vi "手动5界面.vi"(8 "错误输入（无错误）":errorcluster, 10 "界面切换队列":refnum<queue>, 11 "VISA资源名称输入":refnum<visa-resource-name>) -> (0 "错误输出":errorcluster, 3 "VISA资源名称输出":refnum<visa-resource-name>)   [LabVIEW 2018]
panel:
  out "R3":bool
  out "毫秒计时值":u32
  in  "枚举":T1(ring)
  in  "选项卡控件":enum32{"选项卡 1", "选项卡 2"}(tab)
  out "写R14A+读R14B+Z2下降取料":bool
  out "写R144+读R145+Z1下降取料":bool
  out "写R2E+读Y1C+2号吸嘴真空":bool
  out "写R2C+读Y1B+1号吸嘴真空":bool
  out "写R66+读R67+Z2下降取料":bool
  out "写R62+读R63+Z1下降取料":bool
  out "写R1F+读R5F+R2轴旋转定位":bool
  out "写R1C+读R5C+R1轴旋转定位":bool
  out "写R6C+读R6D+Z轴校正位取料":bool
  out "写R64+读R65+XYZ2到2号飞达位":bool
  out "写R60+读R61+XYZ1到飞达位":bool
  out "写R6A+读R6B+Z轴校正位放料":bool
  out "写R3F+读R4F+Z2下降编带":bool
  out "写R3D+读R4D+Z1下降编带":bool
  out "写R148+读R149+Z2下降放料":bool
  out "写R168+读R168+切换+快速":bool
  out "写R142+读R143+Z1下降放料":bool
  out "写R68+读R69+XY到校正位":bool
  out "写R3E+读R4E+XYZ2到2号编带位":bool
  out "写R3C+读R4C+XYZ1到1号编带位":bool
  out "写R146+读R147+XYZ2到烧录位":bool
  out "手动4界面":bool
  out "DDT90356":dbl
  out "DDT90348":dbl
  out "自动界面":bool
  out "手动界面":bool
  out "参数界面":bool
  out "IO界面":bool
  out "产品界面":bool
  out "字符串":string
  out "DDT90352":dbl
  out "DDT90360":dbl
  out "DT1184":T2(ring)
  out "写R0+读R1+手动启动":bool
  out "写R4+读R4+手动停止":bool
  out "写R8+读R9+机器复位":bool
  out "写R80+读R80+报警清除":bool
  out "烧录座手动界面":bool
  out "通讯周期":dbl
  in  "DT62+枚举":enum16{"90度", "180度", "270度"}(ring)
  in  "DT63+枚举":enum16{"90度", "180度", "270度"}(ring)
  out "写R81+读R81+切换+快速":bool
  out "写R140+读141+XYZ1到烧录位":bool
  out "写DT120+指定烧录编号":dbl
  # "X"
  # "Z1"
  # "Z2"
  # "Y"
  # "指定烧录编号"
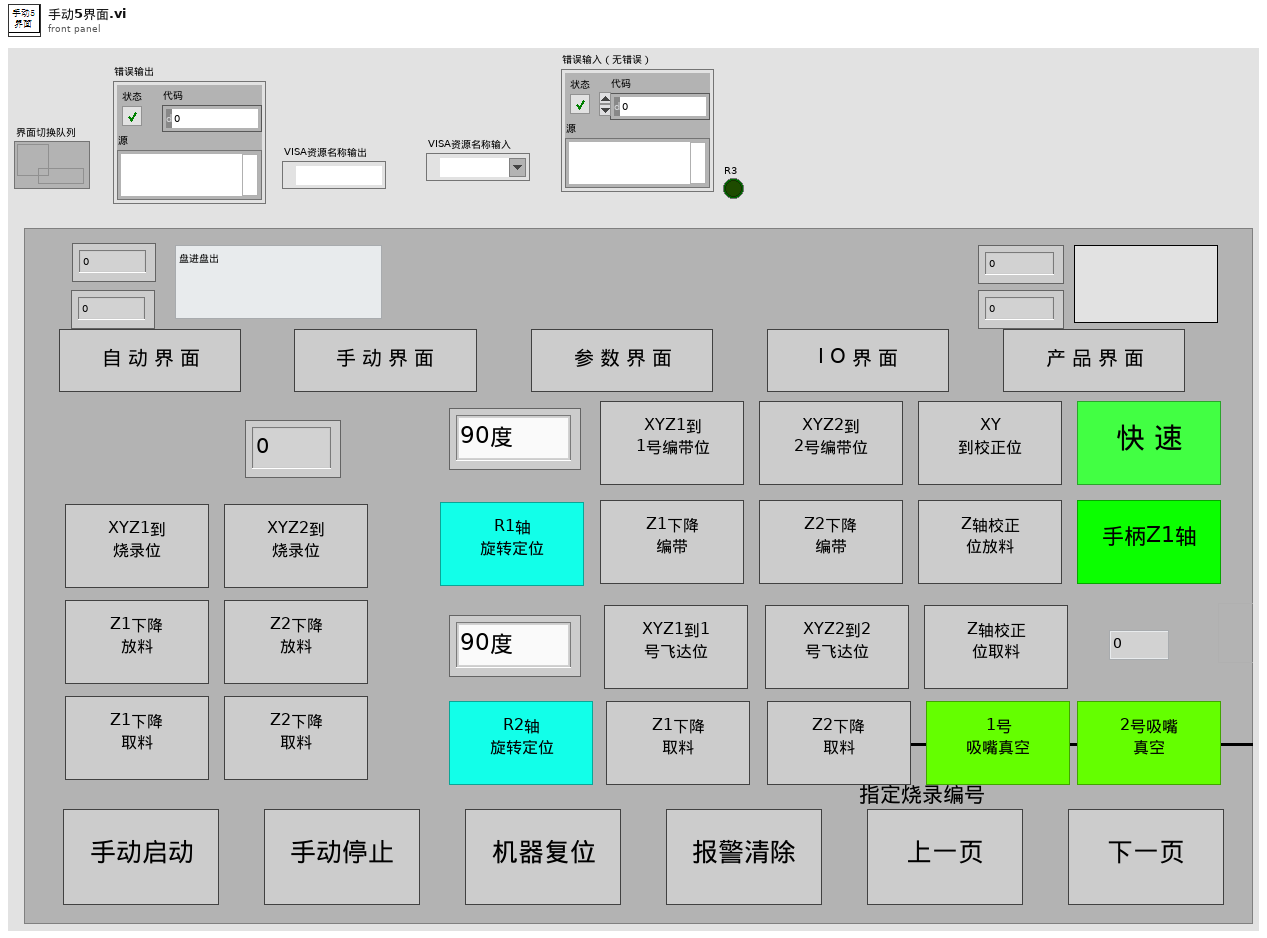
[diagram p1: front panel]
types:
  T1 = enum16{"读初始化", "读R149+8", "读R141+8", "读R4C+8", "读R61+8", "读R77+8", "读R168+8", "读Y1B+8", "读R80+8", "读R69+8", "读R5C+8", "读R9+8", "读R1+8", "读DT770+10", "读DDT604+5", "读DT1184", "读DT62+10", "读DDT90356", "读DDT90348", ""}
  T2 = enum16{"盘进盘出", "卷进卷出", "盘进卷出", "管进盘出", "管进卷出", "卷进盘出", ""}
  T3 = typedef "数据簇.ctl" = cluster{"字符串":string, "数值":i32, "布尔":bool}
  T4 = enum8{"Enabled", "Disabled", "Disabled and Grayed Out"}
  T5 = typedef "lveventtype.ctl" = enum32{"Null", "Timeout", "Annotation Menu Selection", "Annotation Menu Selection?", "App Instance Close", "App Instance Close?", "Autoscale Range Change", "Bookmark Info Change", "Cell Edit", "Cell Edit?", "Cursor Grab", "Cursor Grab?", "Cursor Menu Selection", "Cursor Menu Selection?", "Cursor Move", "Cursor Release", "Data Change", "Direction Change", "Display State Change", "Drag Ended", "Drag Enter", "Drag Leave", "Drag Over", "Drag Source Update", "Drag Starting", "Drag Starting?", "Drop", "Exec State Change", "Key Down", "Key Down?", "Key Repeat", "Key Repeat?", "Key Up", "Listbox Double Click", "Menu Activation?", "Menu Selection (App)", "Menu Selection? (App)", "Menu Selection (User)", "Mouse Down", "Mouse Down?", "Mouse Enter", "Mouse Leave", "Mouse Move", "Mouse Up", "Mouse Wheel", "NI Security User Change (App)", "Pane Size", "Panel Close", "Panel Close?", "Panel Resize", "Plot Attribute Change", "Scale Range Change", "Shortcut Menu Activation?", "Shortcut Menu Selection (App)", "Shortcut Menu Selection? (App)", "Shortcut Menu Selection (User)", "Tree Double Click", "Tree Drag", "Tree Drag?", "Tree Drop", "Tree Drop?", "Tree Item Close", "Tree Item Close?", "Tree Item Open", "Tree Item Open?", "User Event", "Value Change"}
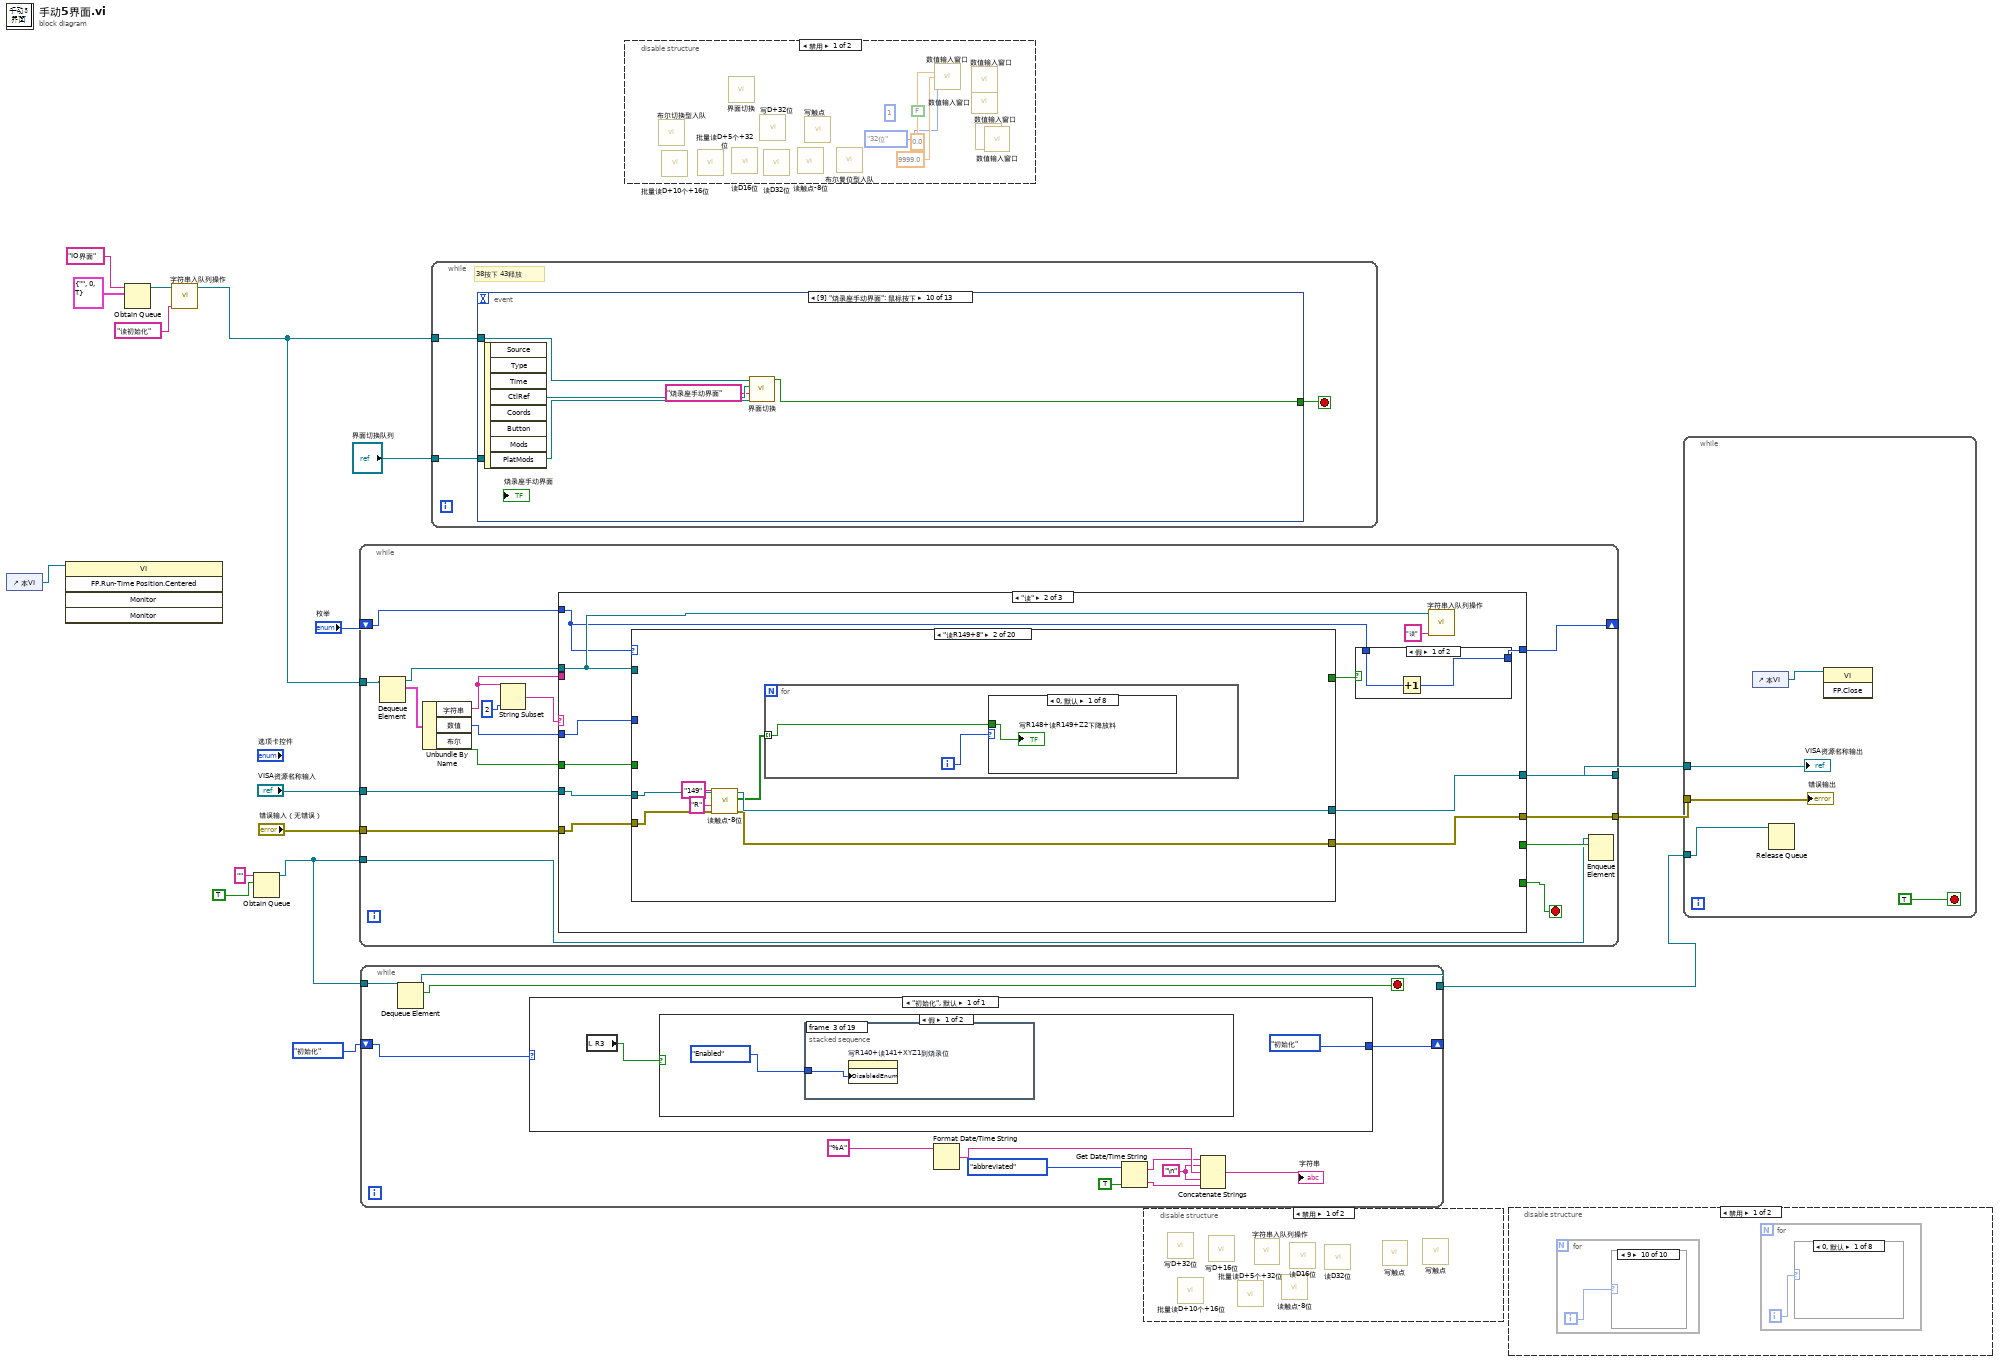
[diagram p0: block diagram]
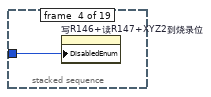
[diagram p4: hidden frame]
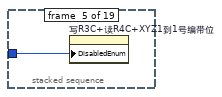
[diagram p5: hidden frame]
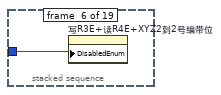
[diagram p6: hidden frame]
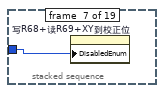
[diagram p7: hidden frame]
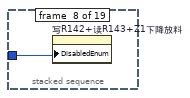
[diagram p8: hidden frame]
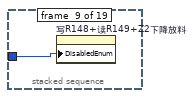
[diagram p9: hidden frame]
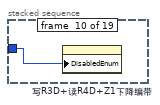
[diagram p10: hidden frame]
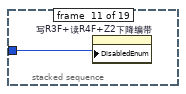
[diagram p11: hidden frame]
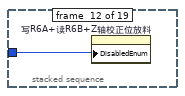
[diagram p12: hidden frame]
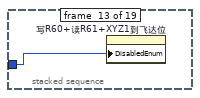
[diagram p13: hidden frame]
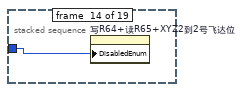
[diagram p14: hidden frame]
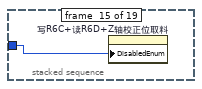
[diagram p15: hidden frame]
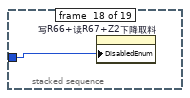
[diagram p18: hidden frame]
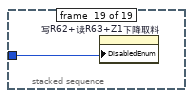
[diagram p19: hidden frame]
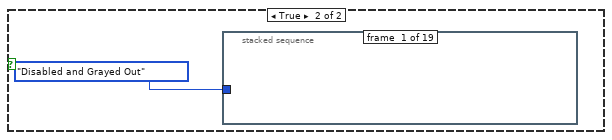
[diagram p20: hidden frame]
diagram:
  n1 = control-ref of="本VI"() -> (w2:refnum<vi>)
  n2 = invoke class="VI" method="FP.Run-Time Position.Centered"(reference=w2) -> ()  [unwired: 4 in, 5 out]
  n3 = Obtain Queue(name (unnamed)="IO界面" ("名称（未命名）"), element data type=T3 {"字符串"="", "数值"=0, "布尔"=TRUE}) -> (queue out=w10:refnum<queue>)  [unwired: 3 in, 2 out]
  n4 = call "字符串入队列操作.vi"("字符消息入队列"="读初始化", "界面切换队列"=w10) -> ("队列输出"=w3:refnum<queue>)  [unwired: 9 in]
  n5 = Obtain Queue(name (unnamed)="" ("名称（未命名）"), element data type=TRUE) -> (queue out=w6:refnum<queue>)  [unwired: 3 in, 2 out]
  n6 = while {
    tunnel: w3 -> [w34]
    tunnel: "VISA资源名称输入" -> [w27]
    tunnel: "错误输入（无错误）" -> [w26]
    tunnel: [w25] -> w12
    tunnel: [w24] -> w11
    shift-right: [w21] -> _
    shift-left: "枚举" -> [w22]
    tunnel: w6 -> [w18]
    stop <- w20 stop-if-true
    n7 = Dequeue Element(queue=w34) -> (queue out=w31:refnum<queue>, element=w33:T3)  [unwired: 2 in, 2 out]
    n8 = Unbundle By Name(w33) -> ("字符串"=w28:string, "数值"=w30:i32, "布尔"=w29:bool)
    n9 = String Subset(string=w28, length (rest)=2 ("长度（剩余）")) -> (substring=w32:string)  [unwired: 1 in]
    n10 = case shown="\"读\"" w32 {
      selector: w32 -> [w37 _ _]
      tunnel: w31 -> [_ w45 w277]
      tunnel: w30 -> [_ w52 w276]
      tunnel: w29 -> [_ w51 w275]
      tunnel: w28 -> [_ _ w269]
      tunnel: w27 -> [w36 w50 w274]
      tunnel: w26 -> [w35 w49 w273]
      tunnel: [w36 w48 w271] -> w25
      tunnel: [w35 w47 w270] -> w24
      tunnel: [_ _ w272] -> w20
      tunnel: w22 -> [_ w43 _]
      tunnel: [_ w42 _] -> w21
      tunnel: [_ _ w267] -> w19
      frame "", Default {
        n11 = Concatenate Strings("无对应消息分支**" ("消息"), w37, "**" ("字符串"), "读写状态机" ("字符串")) -> (w39:string)
        n12 = One Button Dialog(message=w39) -> ()  [unwired: 1 in, 1 out]
      }
      frame "读" {
        n13 = case shown="\"读R149+8\"" w43 {
          tunnel: w45 -> [_ _ _ _ _ _ _ _ _ _ _ _ _ _ _ _ _ _ _ _]
          tunnel: w52 -> [_ _ _ _ _ _ _ _ _ _ _ _ _ _ _ _ _ _ _ _]
          tunnel: w50 -> [w57 w64 w75 w88 w101 w114 w123 w133 w144 w155 w167 w178 w188 w200 w208 w215 w222 w238 w254 w266]
          tunnel: w49 -> [w56 w63 w74 w87 w100 w113 w122 w132 w143 w154 w166 w177 w187 w199 w207 w214 w221 w237 w253 w265]
          tunnel: [w57 w62 w71 w84 w99 w112 w121 w129 w142 w153 w165 w176 w186 w197 w205 w213 w219 w236 w252 w266] -> w48
          tunnel: [w56 w61 w70 w83 w98 w111 w120 w128 w141 w152 w164 w175 w185 w196 w204 w212 w218 w235 w251 w265] -> w47
          tunnel: w51 -> [_ _ _ _ _ _ _ _ _ _ _ _ _ _ _ _ _ _ _ _]
          tunnel: [_ _ _ _ _ _ _ _ _ _ _ _ _ _ _ _ _ _ _ TRUE] -> w44
          frame "读初始化" {
            n14 = Tick Count (ms)() -> (millisecond timer value=→"毫秒计时值":u32)
          }
          frame "读R149+8" {
            n15 = call "读触点-8位.vi"("error out"=w63, "触点类型"="R", "读取起始地址"="149", "VISA resource name out"=w64) -> ("error IO"=w61:errorcluster, "读取布尔数组"=w58:bool[], "VISA resource name out 2"=w62:refnum<visa-resource-name>)  [unwired: 4 in, 1 out]
            n16 = for {
              tunnel: w58 -> [w65] mode=indexing
              i -> [w66]
              n17 = case shown="0, 默认" w66 {
                tunnel: w65 -> [w67 _ w68 _ _ _ _ _]
                frame 0, Default {
                  "写R148+读R149+Z2下降放料" <- w67
                }
                frame 1 {
                }
                frame 2 {
                  "写R14A+读R14B+Z2下降取料" <- w68
                }
                frame 3 {
                }
                frame 4 {
                }
                frame 5 {
                }
                frame 6 {
                }
                frame 7 {
                }
              }
            }
          }
          frame "读R141+8" {
            n18 = call "读触点-8位.vi"("error out"=w74, "触点类型"="R", "读取起始地址"="141", "VISA resource name out"=w75) -> ("error IO"=w70:errorcluster, "读取布尔数组"=w69:bool[], "VISA resource name out 2"=w71:refnum<visa-resource-name>)  [unwired: 4 in, 1 out]
            n19 = for {
              tunnel: w69 -> [w76] mode=indexing
              i -> [w77]
              n20 = case shown="4" w77 {
                tunnel: w76 -> [w78 _ w79 _ w80 _ w81 _]
                frame 0, Default {
                  "写R140+读141+XYZ1到烧录位" <- w78
                }
                frame 1 {
                }
                frame 2 {
                  "写R142+读R143+Z1下降放料" <- w79
                }
                frame 3 {
                }
                frame 4 {
                  "写R144+读R145+Z1下降取料" <- w80
                }
                frame 5 {
                }
                frame 6 {
                  "写R146+读R147+XYZ2到烧录位" <- w81
                }
                frame 7 {
                }
              }
            }
          }
          frame "读R4C+8" {
            n21 = call "读触点-8位.vi"("error out"=w87, "触点类型"="R", "读取起始地址"="4C", "VISA resource name out"=w88) -> ("error IO"=w83:errorcluster, "读取布尔数组"=w82:bool[], "VISA resource name out 2"=w84:refnum<visa-resource-name>)  [unwired: 4 in, 1 out]
            n22 = for {
              tunnel: w82 -> [w89] mode=indexing
              i -> [w90]
              n23 = case shown="3" w90 {
                tunnel: w89 -> [w91 w92 w93 w94 _ _ _ _]
                frame 0, Default {
                  "写R3C+读R4C+XYZ1到1号编带位" <- w91
                }
                frame 1 {
                  "写R3D+读R4D+Z1下降编带" <- w92
                }
                frame 2 {
                  "写R3E+读R4E+XYZ2到2号编带位" <- w93
                }
                frame 3 {
                  "写R3F+读R4F+Z2下降编带" <- w94
                }
                frame 4 {
                }
                frame 5 {
                }
                frame 6 {
                }
                frame 7 {
                }
              }
            }
          }
          frame "读R61+8" {
            n24 = call "读触点-8位.vi"("error out"=w100, "触点类型"="R", "读取起始地址"="61", "VISA resource name out"=w101) -> ("error IO"=w98:errorcluster, "读取布尔数组"=w95:bool[], "VISA resource name out 2"=w99:refnum<visa-resource-name>)  [unwired: 4 in, 1 out]
            n25 = for {
              tunnel: w95 -> [w102] mode=indexing
              i -> [w103]
              n26 = case shown="6" w103 {
                tunnel: w102 -> [w104 _ w105 _ w106 _ w107 _]
                frame 0, Default {
                  "写R60+读R61+XYZ1到飞达位" <- w104
                }
                frame 1 {
                }
                frame 2 {
                  "写R62+读R63+Z1下降取料" <- w105
                }
                frame 3 {
                }
                frame 4 {
                  "写R64+读R65+XYZ2到2号飞达位" <- w106
                }
                frame 5 {
                }
                frame 6 {
                  "写R66+读R67+Z2下降取料" <- w107
                }
                frame 7 {
                }
              }
            }
          }
          frame "读R77+8" {
            n27 = call "读触点-8位.vi"("error out"=w113, "触点类型"="R", "读取起始地址"="77", "VISA resource name out"=w114) -> ("error IO"=w111:errorcluster, "读取布尔数组"=w108:bool[], "VISA resource name out 2"=w112:refnum<visa-resource-name>)  [unwired: 4 in, 1 out]
            n28 = for {
              tunnel: w108 -> [w115] mode=indexing
              i -> [w116]
              n29 = case shown="0, 默认" w116 {
                tunnel: w115 -> [_ _ _ _ _ _ _ _]
                frame 0, Default {
                }
                frame 1 {
                }
                frame 2 {
                }
                frame 3 {
                }
                frame 4 {
                }
                frame 5 {
                }
                frame 6 {
                }
                frame 7 {
                }
              }
            }
          }
          frame "读R168+8" {
            n30 = call "读触点-8位.vi"("error out"=w122, "触点类型"="R", "读取起始地址"="168", "VISA resource name out"=w123) -> ("error IO"=w120:errorcluster, "读取布尔数组"=w117:bool[], "VISA resource name out 2"=w121:refnum<visa-resource-name>)  [unwired: 4 in, 1 out]
            n31 = for {
              tunnel: w117 -> [w124] mode=indexing
              i -> [w125]
              n32 = case shown="0, 默认" w125 {
                tunnel: w124 -> [w126 _ _ _ _ _ _ _]
                frame 0, Default {
                  "写R168+读R168+切换+快速" <- w126
                }
                frame 1 {
                }
                frame 2 {
                }
                frame 3 {
                }
                frame 4 {
                }
                frame 5 {
                }
                frame 6 {
                }
                frame 7 {
                }
              }
            }
          }
          frame "读Y1B+8" {
            n33 = call "读触点-8位.vi"("error out"=w132, "触点类型"="Y", "读取起始地址"="1B", "VISA resource name out"=w133) -> ("error IO"=w128:errorcluster, "读取布尔数组"=w127:bool[], "VISA resource name out 2"=w129:refnum<visa-resource-name>)  [unwired: 4 in, 1 out]
            n34 = for {
              tunnel: w127 -> [w134] mode=indexing
              i -> [w135]
              n35 = case shown="1" w135 {
                tunnel: w134 -> [w136 w137 _ _ _ _ _ _]
                frame 0, Default {
                  "写R2C+读Y1B+1号吸嘴真空" <- w136
                }
                frame 1 {
                  "写R2E+读Y1C+2号吸嘴真空" <- w137
                }
                frame 2 {
                }
                frame 3 {
                }
                frame 4 {
                }
                frame 5 {
                }
                frame 6 {
                }
                frame 7 {
                }
              }
            }
          }
          frame "读R80+8" {
            n36 = call "读触点-8位.vi"("error out"=w143, "触点类型"="R", "读取起始地址"="80", "VISA resource name out"=w144) -> ("error IO"=w141:errorcluster, "读取布尔数组"=w138:bool[], "VISA resource name out 2"=w142:refnum<visa-resource-name>)  [unwired: 4 in, 1 out]
            n37 = for {
              tunnel: w138 -> [w145] mode=indexing
              i -> [w146]
              n38 = case shown="1" w146 {
                tunnel: w145 -> [w147 w148 _ _ _ _ _ _]
                frame 0, Default {
                  "写R80+读R80+报警清除" <- w147
                }
                frame 1 {
                  "写R81+读R81+切换+快速" <- w148
                }
                frame 2 {
                }
                frame 3 {
                }
                frame 4 {
                }
                frame 5 {
                }
                frame 6 {
                }
                frame 7 {
                }
              }
            }
          }
          frame "读R69+8" {
            n39 = call "读触点-8位.vi"("error out"=w154, "触点类型"="R", "读取起始地址"="69", "VISA resource name out"=w155) -> ("error IO"=w152:errorcluster, "读取布尔数组"=w151:bool[], "VISA resource name out 2"=w153:refnum<visa-resource-name>)  [unwired: 4 in, 1 out]
            n40 = for {
              tunnel: w151 -> [w156] mode=indexing
              i -> [w157]
              n41 = case shown="4" w157 {
                tunnel: w156 -> [w158 _ w159 _ w160 _ _ _]
                frame 0, Default {
                  "写R68+读R69+XY到校正位" <- w158
                }
                frame 1 {
                }
                frame 2 {
                  "写R6A+读R6B+Z轴校正位放料" <- w159
                }
                frame 3 {
                }
                frame 4 {
                  "写R6C+读R6D+Z轴校正位取料" <- w160
                }
                frame 5 {
                }
                frame 6 {
                }
                frame 7 {
                }
              }
            }
          }
          frame "读R5C+8" {
            n42 = call "读触点-8位.vi"("error out"=w166, "触点类型"="R", "读取起始地址"="5C", "VISA resource name out"=w167) -> ("error IO"=w164:errorcluster, "读取布尔数组"=w163:bool[], "VISA resource name out 2"=w165:refnum<visa-resource-name>)  [unwired: 4 in, 1 out]
            n43 = for {
              tunnel: w163 -> [w168] mode=indexing
              i -> [w169]
              n44 = case shown="3" w169 {
                tunnel: w168 -> [w170 _ _ w171 _ _ _ _]
                frame 0, Default {
                  "写R1C+读R5C+R1轴旋转定位" <- w170
                }
                frame 1 {
                }
                frame 2 {
                }
                frame 3 {
                  "写R1F+读R5F+R2轴旋转定位" <- w171
                }
                frame 4 {
                }
                frame 5 {
                }
                frame 6 {
                }
                frame 7 {
                }
              }
            }
          }
          frame "读R9+8" {
            n45 = call "读触点-8位.vi"("error out"=w177, "触点类型"="R", "读取起始地址"="9", "VISA resource name out"=w178) -> ("error IO"=w175:errorcluster, "读取布尔数组"=w172:bool[], "VISA resource name out 2"=w176:refnum<visa-resource-name>)  [unwired: 4 in, 1 out]
            n46 = for {
              tunnel: w172 -> [w179] mode=indexing
              i -> [w180]
              n47 = case shown="0, 默认" w180 {
                tunnel: w179 -> [w181 _ _ _ _ _ _ _]
                frame 0, Default {
                  "写R8+读R9+机器复位" <- w181
                }
                frame 1 {
                }
                frame 2 {
                }
                frame 3 {
                }
                frame 4 {
                }
                frame 5 {
                }
                frame 6 {
                }
                frame 7 {
                }
              }
            }
          }
          frame "读R1+8" {
            n48 = call "读触点-8位.vi"("error out"=w187, "触点类型"="R", "读取起始地址"="1", "VISA resource name out"=w188) -> ("error IO"=w185:errorcluster, "读取布尔数组"=w182:bool[], "VISA resource name out 2"=w186:refnum<visa-resource-name>)  [unwired: 4 in, 1 out]
            n49 = for {
              tunnel: w182 -> [w189] mode=indexing
              i -> [w190]
              n50 = case shown="2" w190 {
                tunnel: w189 -> [w191 _ w192 w194 _ _ _ _]
                frame 0, Default {
                  "写R0+读R1+手动启动" <- w191
                }
                frame 1 {
                }
                frame 2 {
                  # "R3"
                  n51 = case shown="假" w192 {
                    selector: w192 -> [w193 _]
                    frame False {
                      "R3" <- w193
                    }
                    frame True {
                      (unwired) T4."Disabled and Grayed Out" ("禁用")
                    }
                  }
                }
                frame 3 {
                  "写R4+读R4+手动停止" <- w194
                }
                frame 4 {
                }
                frame 5 {
                }
                frame 6 {
                }
                frame 7 {
                }
              }
            }
          }
          frame "读DT770+10" {
            n52 = call "批量读D+10个+16位.vi"("error out"=w199, "读取D地址"=770, "VISA resource name out"=w200) -> ("error IO"=w196:errorcluster, "数组"=w195:i32[], "VISA resource name out 2"=w197:refnum<visa-resource-name>)  [unwired: 5 in, 1 out]
            n53 = for {
              tunnel: w195 -> [w201] mode=indexing
              i -> [w202]
              n54 = case shown="0, 默认" w202 {
                tunnel: w201 -> [_ _ _ _ _ _ _ _ _ _]
                frame 0, Default {
                }
                frame 1 {
                }
                frame 2 {
                }
                frame 3 {
                }
                frame 4 {
                }
                frame 5 {
                }
                frame 6 {
                }
                frame 7 {
                }
                frame 8 {
                }
                frame 9 {
                }
              }
            }
          }
          frame "读DDT604+5" {
            n55 = call "批量读D+5个+32位.vi"("error out"=w207, "读取D地址"=604, "VISA resource name out"=w208) -> ("error IO"=w204:errorcluster, "数组"=w203:i32[], "VISA resource name out 2"=w205:refnum<visa-resource-name>)  [unwired: 5 in, 1 out]
            n56 = for {
              tunnel: w203 -> [w209] mode=indexing
              i -> [w210]
              n57 = case shown="0, 默认" w210 {
                tunnel: w209 -> [_ _ _ _ _]
                frame 0, Default {
                }
                frame 1 {
                }
                frame 2 {
                }
                frame 3 {
                }
                frame 4 {
                }
              }
            }
          }
          frame "读DT1184" {
            n58 = call "读D16位.vi"("error out"=w214, "读取D地址"=1184, "VISA resource name out"=w215) -> ("error IO"=w212:errorcluster, "数值"=→"DT1184":u32, "VISA resource name out 2"=w213:refnum<visa-resource-name>)  [unwired: 5 in, 1 out]
          }
          frame "读DT62+10" {
            n59 = call "批量读D+10个+16位.vi"("error out"=w221, "读取D地址"=62, "VISA resource name out"=w222) -> ("error IO"=w218:errorcluster, "数组"=w217:i32[], "VISA resource name out 2"=w219:refnum<visa-resource-name>)  [unwired: 5 in, 1 out]
            n60 = for {
              tunnel: w217 -> [w223] mode=indexing
              i -> [w224]
              n61 = case shown="1" w224 {
                tunnel: w223 -> [w225 w226 _ _ _ _ _ _]
                frame 0, Default {
                  n62 = local write "DT62+枚举"(w225) -> ()
                }
                frame 1 {
                  n63 = local write "DT63+枚举"(w226) -> ()
                }
                frame 2 {
                }
                frame 3 {
                }
                frame 4 {
                }
                frame 5 {
                }
                frame 6 {
                }
                frame 7 {
                }
              }
            }
          }
          frame "读DDT90356" {
            n64 = call "批量读D+5个+32位.vi"("error out"=w237, "读取D地址"=90356, "VISA resource name out"=w238) -> ("error IO"=w235:errorcluster, "数组"=w241:i32[], "VISA resource name out 2"=w236:refnum<visa-resource-name>)  [unwired: 5 in, 1 out]
            n65 = Index Array(array=w241, index #1=0 ("索引"), index #2=2 ("索引")) -> (element #1=w234:i32, element #2=w233:i32)
            n66 = To Double Precision Float(number=w234) -> (double precision float=w232:dbl)
            n67 = To Double Precision Float(number=w233) -> (double precision float=w229:dbl)
            n68 = Divide(x=w232, y=100.0) -> (x/y=→"DDT90356":dbl)
            n69 = Divide(x=w229, y=100.0) -> (x/y=→"DDT90360":dbl)
          }
          frame "读DDT90348" {
            n70 = call "批量读D+5个+32位.vi"("error out"=w253, "读取D地址"=90348, "VISA resource name out"=w254) -> ("error IO"=w251:errorcluster, "数组"=w258:i32[], "VISA resource name out 2"=w252:refnum<visa-resource-name>)  [unwired: 5 in, 1 out]
            n71 = Index Array(array=w258, index #1=0 ("索引"), index #2=2 ("索引")) -> (element #1=w250:i32, element #2=w249:i32)
            n72 = To Double Precision Float(number=w249) -> (double precision float=w244:dbl)
            n73 = To Double Precision Float(number=w250) -> (double precision float=w248:dbl)
            n74 = Divide(x=w244, y=100.0) -> (x/y=→"DDT90352":dbl)
            n75 = Divide(x=w248, y=100.0) -> (x/y=→"DDT90348":dbl)
          }
          frame "" {
            n76 = local read "毫秒计时值"() -> (w262:u32)
            n77 = Tick Count (ms)() -> (millisecond timer value=w263:u32)
            n78 = Subtract(x=w263, y=w262) -> (x-y=w261:u32)
            n79 = Divide(x=w261, y=u32 1000) -> (x/y=→"通讯周期":dbl)
          }
        }
        n80 = case shown="假" w44 {
          tunnel: w43 -> [w54 _]
          tunnel: [w53 _] -> w42
          frame False {
            n81 = Increment(x=w54) -> (x+1=w53:T1)
          }
          frame True {
          }
        }
        n82 = call "字符串入队列操作.vi"("字符消息入队列"="读", "界面切换队列"=w45) -> ()  [unwired: 9 in, 1 out]
      }
      frame "写" {
        n83 = call "状态匹配.vi"("输入状态"=w269) -> ("输出状态"=w268:string)  [unwired: 10 in]
        n84 = case shown="\"写R\"" w268 {
          selector: w268 -> [w280 _ _ _ _]
          tunnel: w277 -> [_ _ _ _ w320]
          tunnel: w276 -> [_ w286 w303 _ _]
          tunnel: w275 -> [_ _ _ w314 _]
          tunnel: w274 -> [w279 w296 w307 w319 w325]
          tunnel: w273 -> [w278 w295 w306 w318 w324]
          tunnel: [_ _ _ _ w323] -> w272
          tunnel: [w279 w294 w305 w317 w325] -> w271
          tunnel: [w278 w293 w304 w316 w324] -> w270
          tunnel: w269 -> [_ w285 w297 w308 _]
          tunnel: [_ _ _ _ w323] -> w267
          frame "", Default {
            n85 = Concatenate Strings("无对应消息分支**" ("消息"), w280, "**" ("字符串"), "写状态机" ("字符串")) -> (w284:string)
            n86 = One Button Dialog(message=w284) -> ()  [unwired: 1 in, 1 out]
          }
          frame "写DT" {
            n87 = String Length(string=w285) -> (length=w291:i32)
            n88 = Subtract(x=w291, y=4) -> (x-y=w289:i32)
            n89 = String Subset(string=w285, offset (0)=4 ("偏移量(0)"), length (rest)=w289) -> (substring=w288:string)
            n90 = Decimal String To Number(string=w288) -> (number=w287:i32)  [unwired: 2 in, 1 out]
            n91 = call "写D+16位.vi"("error out"=w295, "输入数值"=w286, "输入地址D"=w287, "VISA resource name out"=w296) -> ("error out 2"=w293:errorcluster, "VISA resource name out 2"=w294:refnum<visa-resource-name>)  [unwired: 3 in, 3 out]
          }
          frame "写DDT" {
            n92 = String Length(string=w297) -> (length=w301:i32)
            n93 = Subtract(x=w301, y=5) -> ()  [unwired: 1 out]
            n94 = String Subset(string=w297, offset (0)=5 ("偏移量(0)")) -> (substring=w298:string)  [unwired: 1 in]
            n95 = Decimal String To Number(string=w298) -> (number=w299:i32)  [unwired: 2 in, 1 out]
            n96 = call "写D+32位.vi"("error out"=w306, "输入数值"=w303, "输入地址D"=w299, "VISA resource name out"=w307) -> ("error out 2"=w304:errorcluster, "VISA resource name out 2"=w305:refnum<visa-resource-name>)  [unwired: 4 in, 2 out]
          }
          frame "写R" {
            n97 = String Length(string=w308) -> (length=w312:i32)
            n98 = Subtract(x=w312, y=3) -> (x-y=w310:i32)
            n99 = String Subset(string=w308, offset (0)=3 ("偏移量(0)"), length (rest)=w310) -> (substring=w309:string)
            n100 = call "写触点.vi"("布尔"=w314, "error out"=w318, "触点类型"="R", "写入起始地址"=w309, "VISA resource name out"=w319) -> ("error IO"=w316:errorcluster, "VISA resource name out 2"=w317:refnum<visa-resource-name>)  [unwired: 4 in, 1 out]
          }
          frame "写退出" {
            w323 = TRUE
            n101 = Flush Queue(queue=w320) -> (queue out=w321:refnum<queue>, error out=w322:errorcluster)  [unwired: 1 in, 1 out]
            n102 = Release Queue(queue=w321, error in (no error)=w322) -> ()  [unwired: 1 in, 3 out]
          }
        }
      }
    }
    n103 = Enqueue Element(queue=w18, element=w19) -> ()  [unwired: 2 in, 3 out]
  }
  n104 = while {
    shift-right: [w337] -> _
    shift-left: enum16{"初始化"}."初始化" -> [w338]
    tunnel: w6 -> [w336]
    tunnel: [w334] -> w5
    stop <- w335 stop-if-true
    w328 = "\n"
    n105 = Dequeue Element(queue=w336) -> (queue out=w334:refnum<queue>, element=w335:bool)  [unwired: 2 in, 2 out]
    n106 = case shown="\"初始化\", 默认" w338 {
      tunnel: [enum16{"初始化"}."初始化"] -> w337
      frame "初始化", Default {
        n107 = local read "R3"() -> (w339:bool)
        n108 = case shown="假" w339 {
          frame False {
            n109 = stacked-sequence {
              tunnel: T4."Enabled" ("禁用") -> [_ _ w342 w343 w344 w345 w346 w347 w348 w349 w350 w351 w352 w353 w354 _ _ w355 w356]
              frame #0 {
              }
              frame #1 {
              }
              frame #2 {
                n110 = property on="写R140+读141+XYZ1到烧录位" class="Bool"("DisabledEnum"=w342) -> ()  [unwired: 2 in, 2 out]
              }
              frame #3 {
                n111 = property on="写R146+读R147+XYZ2到烧录位" class="Bool"("DisabledEnum"=w343) -> ()  [unwired: 2 in, 2 out]
              }
              frame #4 {
                n112 = property on="写R3C+读R4C+XYZ1到1号编带位" class="Bool"("DisabledEnum"=w344) -> ()  [unwired: 2 in, 2 out]
              }
              frame #5 {
                n113 = property on="写R3E+读R4E+XYZ2到2号编带位" class="Bool"("DisabledEnum"=w345) -> ()  [unwired: 2 in, 2 out]
              }
              frame #6 {
                n114 = property on="写R68+读R69+XY到校正位" class="Bool"("DisabledEnum"=w346) -> ()  [unwired: 2 in, 2 out]
              }
              frame #7 {
                n115 = property on="写R142+读R143+Z1下降放料" class="Bool"("DisabledEnum"=w347) -> ()  [unwired: 2 in, 2 out]
              }
              frame #8 {
                n116 = property on="写R148+读R149+Z2下降放料" class="Bool"("DisabledEnum"=w348) -> ()  [unwired: 2 in, 2 out]
              }
              frame #9 {
                n117 = property on="写R3D+读R4D+Z1下降编带" class="Bool"("DisabledEnum"=w349) -> ()  [unwired: 2 in, 2 out]
              }
              frame #10 {
                n118 = property on="写R3F+读R4F+Z2下降编带" class="Bool"("DisabledEnum"=w350) -> ()  [unwired: 2 in, 2 out]
              }
              frame #11 {
                n119 = property on="写R6A+读R6B+Z轴校正位放料" class="Bool"("DisabledEnum"=w351) -> ()  [unwired: 2 in, 2 out]
              }
              frame #12 {
                n120 = property on="写R60+读R61+XYZ1到飞达位" class="Bool"("DisabledEnum"=w352) -> ()  [unwired: 2 in, 2 out]
              }
              frame #13 {
                n121 = property on="写R64+读R65+XYZ2到2号飞达位" class="Bool"("DisabledEnum"=w353) -> ()  [unwired: 2 in, 2 out]
              }
              frame #14 {
                n122 = property on="写R6C+读R6D+Z轴校正位取料" class="Bool"("DisabledEnum"=w354) -> ()  [unwired: 2 in, 2 out]
              }
              frame #15 {
              }
              frame #16 {
              }
              frame #17 {
                n123 = property on="写R66+读R67+Z2下降取料" class="Bool"("DisabledEnum"=w355) -> ()  [unwired: 2 in, 2 out]
              }
              frame #18 {
                n124 = property on="写R62+读R63+Z1下降取料" class="Bool"("DisabledEnum"=w356) -> ()  [unwired: 2 in, 2 out]
              }
            }
          }
          frame True {
            n125 = stacked-sequence {
              tunnel: T4."Disabled and Grayed Out" ("禁用") -> [_ _ w358 w359 w360 w361 w362 w363 w364 w365 w366 w367 w368 w369 w370 _ _ w371 w372]
              frame #0 {
              }
              frame #1 {
              }
              frame #2 {
                n126 = property on="写R140+读141+XYZ1到烧录位" class="Bool"("DisabledEnum"=w358) -> ()  [unwired: 2 in, 2 out]
              }
              frame #3 {
                n127 = property on="写R146+读R147+XYZ2到烧录位" class="Bool"("DisabledEnum"=w359) -> ()  [unwired: 2 in, 2 out]
              }
              frame #4 {
                n128 = property on="写R3C+读R4C+XYZ1到1号编带位" class="Bool"("DisabledEnum"=w360) -> ()  [unwired: 2 in, 2 out]
              }
              frame #5 {
                n129 = property on="写R3E+读R4E+XYZ2到2号编带位" class="Bool"("DisabledEnum"=w361) -> ()  [unwired: 2 in, 2 out]
              }
              frame #6 {
                n130 = property on="写R68+读R69+XY到校正位" class="Bool"("DisabledEnum"=w362) -> ()  [unwired: 2 in, 2 out]
              }
              frame #7 {
                n131 = property on="写R142+读R143+Z1下降放料" class="Bool"("DisabledEnum"=w363) -> ()  [unwired: 2 in, 2 out]
              }
              frame #8 {
                n132 = property on="写R148+读R149+Z2下降放料" class="Bool"("DisabledEnum"=w364) -> ()  [unwired: 2 in, 2 out]
              }
              frame #9 {
                n133 = property on="写R3D+读R4D+Z1下降编带" class="Bool"("DisabledEnum"=w365) -> ()  [unwired: 2 in, 2 out]
              }
              frame #10 {
                n134 = property on="写R3F+读R4F+Z2下降编带" class="Bool"("DisabledEnum"=w366) -> ()  [unwired: 2 in, 2 out]
              }
              frame #11 {
                n135 = property on="写R6A+读R6B+Z轴校正位放料" class="Bool"("DisabledEnum"=w367) -> ()  [unwired: 2 in, 2 out]
              }
              frame #12 {
                n136 = property on="写R60+读R61+XYZ1到飞达位" class="Bool"("DisabledEnum"=w368) -> ()  [unwired: 2 in, 2 out]
              }
              frame #13 {
                n137 = property on="写R64+读R65+XYZ2到2号飞达位" class="Bool"("DisabledEnum"=w369) -> ()  [unwired: 2 in, 2 out]
              }
              frame #14 {
                n138 = property on="写R6C+读R6D+Z轴校正位取料" class="Bool"("DisabledEnum"=w370) -> ()  [unwired: 2 in, 2 out]
              }
              frame #15 {
              }
              frame #16 {
              }
              frame #17 {
                n139 = property on="写R66+读R67+Z2下降取料" class="Bool"("DisabledEnum"=w371) -> ()  [unwired: 2 in, 2 out]
              }
              frame #18 {
                n140 = property on="写R62+读R63+Z1下降取料" class="Bool"("DisabledEnum"=w372) -> ()  [unwired: 2 in, 2 out]
              }
            }
          }
        }
      }
    }
    n141 = Format Date/Time String(time format string (%c)="%A" ("时间格式字符串(%c)")) -> (date/time string=w332:string)  [unwired: 2 in]
    n142 = Get Date/Time String(date format (0)=enum16{"short", "long", "abbreviated"}."abbreviated" ("日期格式(0)"), want seconds? (F)=TRUE ("需要秒？(F)")) -> (date string=w330:string, time string=w333:string)  [unwired: 1 in]
    n143 = Concatenate Strings(w330, w328, w332, w328, w333) -> (→"字符串":string)
  }
  n144 = while {
    tunnel: w3 -> [w374]
    tunnel: "界面切换队列" -> [w373]
    stop <- w375 stop-if-true
    # "38按下 43释放"
    n145 = event shown="[9] \"烧录座手动界面\": 鼠标按下" {
      selector: _ -> [_ _ _ _ _ _ _ _ _ _ _ _ _]
      dyn-events: _ -> [_ _ _ _ _ _ _ _ _ _ _ _ _]
      timeout: _ -> [_ _ _ _ _ _ _ _ _ _ _ _ _]
      tunnel: [w376 w383 _ _ _ _ w406 w411 w416 w421 w426 _ w433] -> w375
      tunnel: w374 -> [w380 w385 w388 w392 w402 w405 w410 w415 w420 w425 w430 _ w432]
      tunnel: w373 -> [w379 w384 _ _ _ _ w409 w414 w419 w424 w429 _ w431]
      event "IO界面": Mouse Down {
        n146 = event-data() -> ("CtlRef"=w378:refnum<vi>)  [unwired: 1 in, 7 out]
        n147 = call "界面切换.vi"("界面切换队列输入"=w379, "切换界面名称输入"="IO界面", "Bool引用句柄"=w378, "状态转移输入"=w380) -> ("布尔"=w376:bool)  [unwired: 7 in]
      }
      event "参数界面": Mouse Down {
        n148 = event-data() -> ("CtlRef"=w382:refnum<vi>)  [unwired: 1 in, 7 out]
        n149 = call "界面切换.vi"("界面切换队列输入"=w384, "切换界面名称输入"="参数界面", "Bool引用句柄"=w382, "状态转移输入"=w385) -> ("布尔"=w383:bool)  [unwired: 7 in]
      }
      event "DT62+枚举": Value Change {
        n150 = event-data() -> ("NewVal"=w387:enum16{"90度", "180度", "270度"})  [unwired: 1 in, 5 out]
        n151 = call "字符串入队列操作.vi"("字符消息入队列"="写DT62", "数值"=w387, "界面切换队列"=w388) -> ()  [unwired: 8 in, 1 out]
      }
      event "写R14A+读R14B+Z2下降取料", "写R4+读R4+手动停止", "写R8+读R9+机器复位", "写R80+读R80+报警清除", "写R140+读141+XYZ1到烧录位", "写R146+读R147+XYZ2到烧录位", "写R3C+读R4C+XYZ1到1号编带位", "写R3E+读R4E+XYZ2到2号编带位", "写R68+读R69+XY到校正位", "写R142+读R143+Z1下降放料", "写R148+读R149+Z2下降放料", "写R3D+读R4D+Z1下降编带", "写R3F+读R4F+Z2下降编带", "写R6A+读R6B+Z轴校正位放料", "写R60+读R61+XYZ1到飞达位", "写R64+读R65+XYZ2到2号飞达位", "写R6C+读R6D+Z轴校正位取料", "写R1C+读R5C+R1轴旋转定位", "写R1F+读R5F+R2轴旋转定位", "写R62+读R63+Z1下降取料", "写R66+读R67+Z2下降取料", "写R2C+读Y1B+1号吸嘴真空", "写R2E+读Y1C+2号吸嘴真空", "写R144+读R145+Z1下降取料": Mouse Down; "写R0+读R1+手动启动", "写R4+读R4+手动停止", "写R8+读R9+机器复位", "写R80+读R80+报警清除", "写R140+读141+XYZ1到烧录位", "写R146+读R147+XYZ2到烧录位", "写R3C+读R4C+XYZ1到1号编带位", "写R3E+读R4E+XYZ2到2号编带位", "写R68+读R69+XY到校正位", "写R142+读R143+Z1下降放料", "写R148+读R149+Z2下降放料", "写R3D+读R4D+Z1下降编带", "写R3F+读R4F+Z2下降编带", "写R6A+读R6B+Z轴校正位放料", "写R60+读R61+XYZ1到飞达位", "写R64+读R65+XYZ2到2号飞达位", "写R6C+读R6D+Z轴校正位取料", "写R1C+读R5C+R1轴旋转定位", "写R1F+读R5F+R2轴旋转定位", "写R62+读R63+Z1下降取料", "写R66+读R67+Z2下降取料", "写R2C+读Y1B+1号吸嘴真空", "写R2E+读Y1C+2号吸嘴真空", "写R144+读R145+Z1下降取料", "写R14A+读R14B+Z2下降取料": Mouse Up {
        n152 = event-data() -> ("Type"=w390:T5, "CtlRef"=w395:refnum<vi>)  [unwired: 1 in, 6 out]
        n153 = property class="Bool"(reference=w395) -> (reference out=w391:refnum<vi>, "Label.Text"=w394:string)  [unwired: 1 in, 1 out]
        n154 = Match Pattern(string=w394, regular expression="+" ("正则表达式")) -> (before substring=w389:string)  [unwired: 1 in, 3 out]
        n155 = call "布尔复位型入队.vi"("队列输入"=w392, "数值"=w390, "控件引用"=w391, "字符消息入队列"=w389) -> ()  [unwired: 2 in, 3 out]
      }
      event "写R81+读R81+切换+快速", "写R168+读R168+切换+快速": Mouse Down {
        n156 = event-data() -> ("CtlRef"=w401:refnum<vi>)  [unwired: 1 in, 7 out]
        n157 = property class="Bool"(reference=w401) -> (reference out=w396:refnum<vi>, "Label.Text"=w400:string)  [unwired: 1 in, 1 out]
        n158 = Match Pattern(string=w400, regular expression="+" ("正则表达式")) -> (before substring=w398:string)  [unwired: 1 in, 3 out]
        n159 = call "布尔切换型入队.vi"("字符串"=w398, "true启用入队"=TRUE, "控件引用"=w396, "消息入队列"=w402) -> ()  [unwired: 8 in]
      }
      event "DT63+枚举": Value Change {
        n160 = event-data() -> ("NewVal"=w404:enum16{"90度", "180度", "270度"})  [unwired: 1 in, 5 out]
        n161 = call "字符串入队列操作.vi"("字符消息入队列"="写DT63", "数值"=w404, "界面切换队列"=w405) -> ()  [unwired: 8 in, 1 out]
      }
      event "产品界面": Mouse Down {
        n162 = event-data() -> ("CtlRef"=w408:refnum<vi>)  [unwired: 1 in, 7 out]
        n163 = call "界面切换.vi"("界面切换队列输入"=w409, "切换界面名称输入"="产品界面", "Bool引用句柄"=w408, "状态转移输入"=w410) -> ("布尔"=w406:bool)  [unwired: 7 in]
      }
      event "手动界面": Mouse Down {
        n164 = event-data() -> ("CtlRef"=w413:refnum<vi>)  [unwired: 1 in, 7 out]
        n165 = call "界面切换.vi"("界面切换队列输入"=w414, "切换界面名称输入"="手动界面", "Bool引用句柄"=w413, "状态转移输入"=w415) -> ("布尔"=w411:bool)  [unwired: 7 in]
      }
      event "手动4界面": Mouse Down {
        n166 = event-data() -> ("CtlRef"=w418:refnum<vi>)  [unwired: 1 in, 7 out]
        n167 = call "界面切换.vi"("界面切换队列输入"=w419, "切换界面名称输入"="手动3界面", "Bool引用句柄"=w418, "状态转移输入"=w420) -> ("布尔"=w416:bool)  [unwired: 7 in]
      }
      event "烧录座手动界面": Mouse Down {
        n168 = event-data() -> ("CtlRef"=w423:refnum<vi>)  [unwired: 1 in, 7 out]
        n169 = call "界面切换.vi"("界面切换队列输入"=w424, "切换界面名称输入"="烧录座手动界面", "Bool引用句柄"=w423, "状态转移输入"=w425) -> ("布尔"=w421:bool)  [unwired: 7 in]
      }
      event "自动界面": Mouse Down {
        n170 = event-data() -> ("CtlRef"=w428:refnum<vi>)  [unwired: 1 in, 7 out]
        n171 = call "界面切换.vi"("界面切换队列输入"=w429, "切换界面名称输入"="自动界面", "Bool引用句柄"=w428, "状态转移输入"=w430) -> ("布尔"=w426:bool)  [unwired: 7 in]
      }
      event Timeout {
        n172 = event-data() -> ()  [unwired: 1 in, 3 out]
      }
      event Panel Close? {
        n173 = event-data() -> ()  [unwired: 1 in, 4 out]
        n174 = Two Button Dialog(message="确定退出程序？" ("消息")) -> (T button?=w434:bool)  [unwired: 2 in]
        n175 = case shown="真" w434 {
          tunnel: [_ TRUE] -> w433
          tunnel: w432 -> [_ w439]
          tunnel: w431 -> [_ w438]
          frame False {
          }
          frame True {
            n176 = call "字符串入队列操作.vi"("字符消息入队列"="退出", "界面切换队列"=w438) -> ()  [unwired: 9 in, 1 out]
            n177 = call "字符串入队列操作.vi"("字符消息入队列"="写退出", "界面切换队列"=w439) -> ()  [unwired: 9 in, 1 out]
          }
        }
        n178 = event-data("Discard?"=TRUE ("放弃？")) -> ()  [unwired: 1 in, 1 out]
      }
    }
  }
  n179 = disable-structure shown="禁用" {
    frame Disabled {
      (unwired) u32 1 ("转换比例")
      (unwired) FALSE ("忽略数值上下限")
      n180 = call "布尔切换型入队.vi"() -> ()  [unwired: 12 in]
      n181 = call "批量读D+10个+16位.vi"() -> ()  [unwired: 8 in, 4 out]
      n182 = call "批量读D+5个+32位.vi"() -> ()  [unwired: 8 in, 4 out]
      n183 = call "界面切换.vi"() -> ()  [unwired: 11 in, 1 out]
      n184 = call "读D16位.vi"() -> ()  [unwired: 8 in, 4 out]
      n185 = call "写D+32位.vi"() -> ()  [unwired: 8 in, 4 out]
      n186 = call "读D32位.vi"() -> ()  [unwired: 9 in, 3 out]
      n187 = call "读触点-8位.vi"() -> ()  [unwired: 8 in, 4 out]
      n188 = call "写触点.vi"() -> ()  [unwired: 9 in, 3 out]
      n189 = call "布尔复位型入队.vi"() -> ()  [unwired: 6 in, 3 out]
      n190 = call "数值输入窗口.vi"("输入下限"=0.0, "输入上限"=9999.0, "数据类型"=enum16{"32位", "16位"}."32位") -> ("转换比例"=w445:u32)  [unwired: 9 in, 3 out]
      n191 = call "数值输入窗口.vi"() -> ()  [unwired: 13 in, 3 out]
      n192 = call "数值输入窗口.vi"() -> ()  [unwired: 13 in, 3 out]
      n193 = call "数值输入窗口.vi"() -> ()  [unwired: 13 in, 3 out]
      n194 = call "数值输入窗口.vi"() -> ()  [unwired: 13 in, 3 out]
    }
    frame Enabled {
    }
  }
  n195 = disable-structure shown="禁用" {
    frame Disabled {
      n196 = call "写D+32位.vi"() -> ()  [unwired: 8 in, 4 out]
      n197 = call "批量读D+10个+16位.vi"() -> ()  [unwired: 8 in, 4 out]
      n198 = call "写D+16位.vi"() -> ()  [unwired: 7 in, 5 out]
      n199 = call "批量读D+5个+32位.vi"() -> ()  [unwired: 8 in, 4 out]
      n200 = call "字符串入队列操作.vi"() -> ()  [unwired: 11 in, 1 out]
      n201 = call "读触点-8位.vi"() -> ()  [unwired: 8 in, 4 out]
      n202 = call "读D16位.vi"() -> ()  [unwired: 8 in, 4 out]
      n203 = call "读D32位.vi"() -> ()  [unwired: 9 in, 3 out]
      n204 = call "写触点.vi"() -> ()  [unwired: 9 in, 3 out]
      n205 = call "写触点.vi"() -> ()  [unwired: 9 in, 3 out]
    }
    frame Enabled {
    }
  }
  n206 = disable-structure shown="禁用" {
    frame Disabled {
      n207 = for {
        i -> [w447]
        n208 = case shown="9" w447 {
          frame 0, Default {
          }
          frame 1 {
          }
          frame 2 {
          }
          frame 3 {
          }
          frame 4 {
          }
          frame 5 {
          }
          frame 6 {
          }
          frame 7 {
          }
          frame 8 {
          }
          frame 9 {
          }
        }
      }
      n209 = for {
        i -> [w446]
        n210 = case shown="0, 默认" w446 {
          frame 0, Default {
          }
          frame 1 {
          }
          frame 2 {
          }
          frame 3 {
          }
          frame 4 {
          }
          frame 5 {
          }
          frame 6 {
          }
          frame 7 {
          }
        }
      }
    }
    frame Enabled {
    }
  }
  n211 = while {
    tunnel: w12 -> [w450]
    tunnel: w11 -> [w449]
    tunnel: w5 -> [w448]
    stop <- TRUE stop-if-true
    n212 = control-ref of="本VI"() -> (w451:refnum<vi>)
    n213 = Release Queue(queue=w448) -> ()  [unwired: 2 in, 3 out]
    n214 = invoke class="VI" method="FP.Close"(reference=w451) -> ()  [unwired: 2 in, 3 out]
    "VISA资源名称输出" <- w450
    "错误输出" <- w449
  }
